vi "系统 interface write.vi"(11 "与系统交互":T1={"运行模式"=enum."维护模式", "运行间隔"=4, "流程运行中"=FALSE, "自动运行启动参数"={"氨氮"=FALSE, "总磷"=FALSE, "总氮"=FALSE, "多参数"=FALSE, "CODmn"=FALSE, "CODCr"=FALSE, "氟化物"=FALSE, "超标留样"=FALSE, "重金属"=FALSE, "挥发酚"=FALSE}, "SYSTEM Interface.总磷总氮类型"=enum."单模块", "多参数运行间隔"=4, "配水时间"=0.0, "沉淀时间"=0.0, "清洗时间"=0.0, "关键参数改变"=FALSE, "温度告警"=FALSE, "湿度告警"=FALSE, "烟感告警"=FALSE, "水浸告警"=FALSE, "开门告警"=FALSE, "SystemTask"=enum."停机", "PumpState"=enum."--", "除藻选择"=enum."不开除藻", "报警信息"=enum."无报警", "软件升级"=FALSE} {"多参数运行间隔" min=1 max=24; "运行间隔" min=1 max=24}) -> ()   [LabVIEW 2016, in "MB SLAVE.lvlib"]
uses:
  MB SLAVE.lvlib
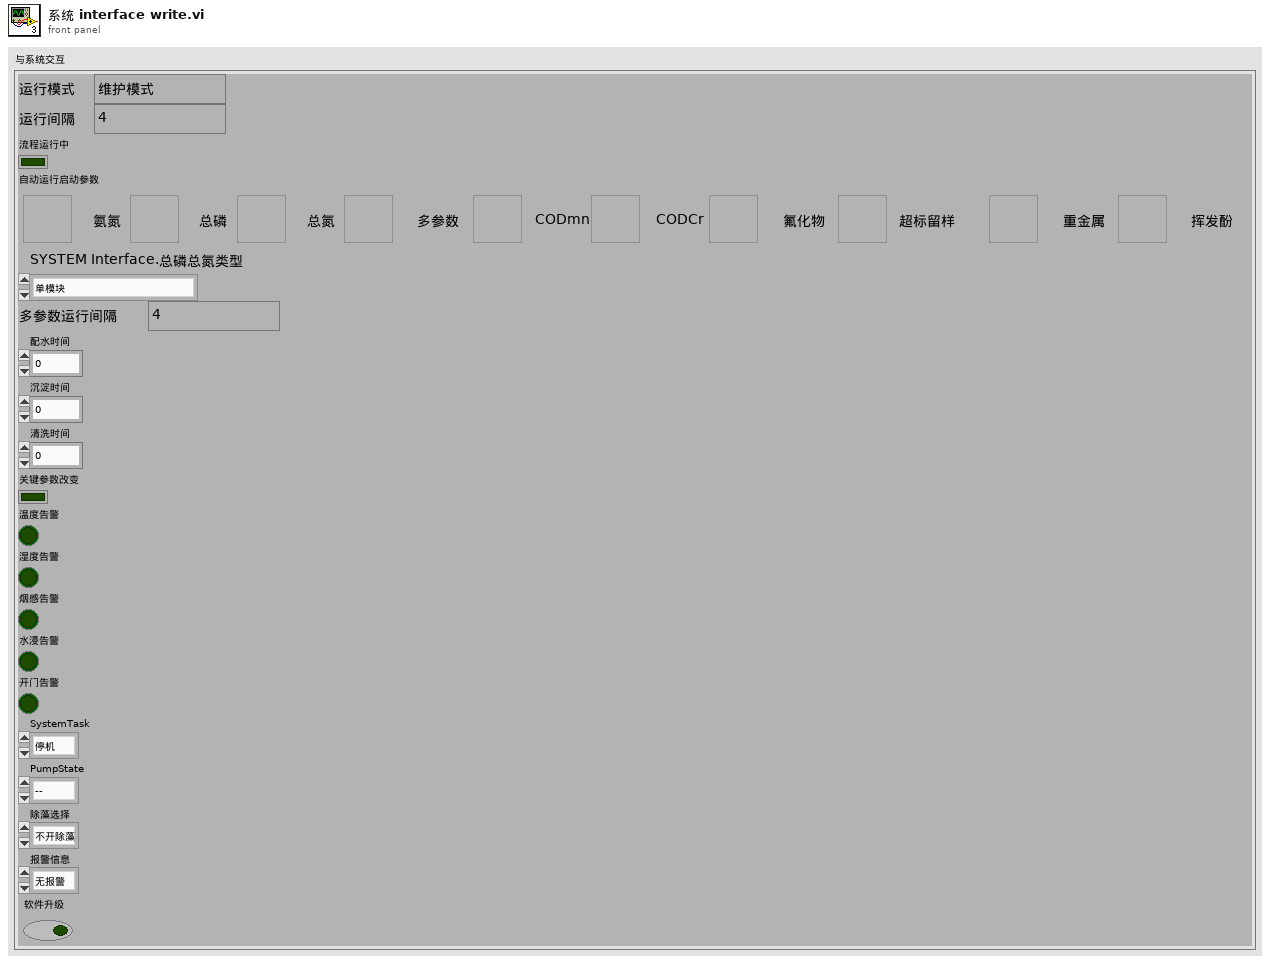
[diagram p1: front panel]
types:
  T1 = typedef "系统交互.ctl" = cluster{"运行模式":enum16{"维护模式", "常规模式", "应急模式", "质控模式", "性能测试"}, "运行间隔":i16, "流程运行中":bool, "自动运行启动参数":T2, "SYSTEM Interface.总磷总氮类型":enum16{"单模块", "总磷总氮二合一模块", "氨氮总磷二合一模块"}, "多参数运行间隔":i16, "配水时间":dbl, "沉淀时间":dbl, "清洗时间":dbl, "关键参数改变":bool, "温度告警":bool, "湿度告警":bool, "烟感告警":bool, "水浸告警":bool, "开门告警":bool, "SystemTask":enum16{"停机", "待机", "调试", "水样采集", "沉沙", "进样", "仪表测试分析", "反吹", "清洗", "除藻"}, "PumpState":enum16{"--", "只用泵1", "只用泵2", "双泵交替"}, "除藻选择":enum16{"不开除藻", "开除藻"}, "报警信息":enum16{"无报警", "断电报警", "采样管理欠压（源水泵故障）", "进样管路欠压（进样泵/增加泵故障）"}, "软件升级":bool}
  T2 = typedef "启动参数.ctl" = cluster{"氨氮":bool, "总磷":bool, "总氮":bool, "多参数":bool, "CODmn":bool, "CODCr":bool, "氟化物":bool, "超标留样":bool, "重金属":bool, "挥发酚":bool}
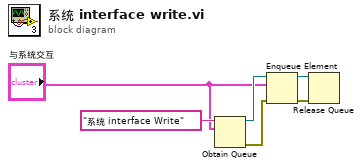
[diagram p0: block diagram]
diagram:
  n1 = Obtain Queue(name (unnamed)="系统 interface Write" ("写入方名称"), element data type="与系统交互") -> (queue out=w6:refnum<queue>, error out=w5:errorcluster)  [unwired: 3 in, 1 out]
  n2 = Enqueue Element(queue=w6, element="与系统交互", error in (no error)=w5) -> (queue out=w3:refnum<queue>, error out=w2:errorcluster)  [unwired: 1 in, 1 out]
  n3 = Release Queue(queue=w3, error in (no error)=w2) -> ()  [unwired: 1 in, 3 out]
